vi "niDTS BT INSTR RX Abort.vi"(8 "error in (no error)":errorcluster, 10 "Driver Instance":i32, 11 "niDTS BT INSTR RX in":refnum<class "niDTS BT INSTR RX.lvclass">) -> (0 "error out":errorcluster, 3 "niDTS BT INSTR RX out":refnum<class "niDTS BT INSTR RX.lvclass">)   [LabVIEW 2015, in "niDTS BT.lvlib" / "niDTS BT INSTR RX.lvclass"]
uses:
  niDTS BT INSTR RX.lvclass
  RiviInstDriver/niRfsgBT/Objects/niRfsgBt.lvclass
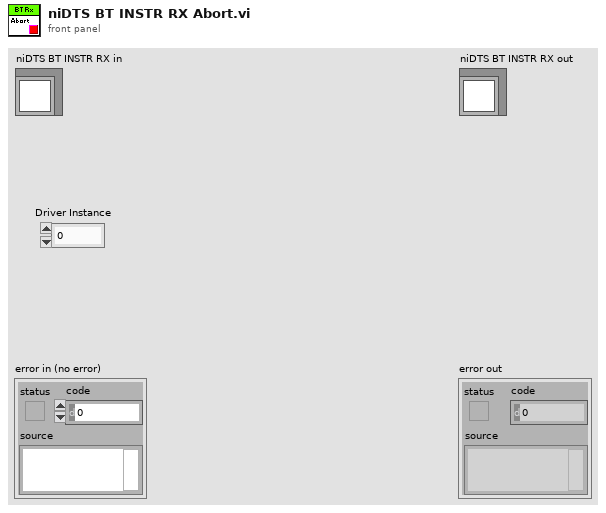
[diagram p1: front panel]
types:
  T1 = typedef "niRfsgBT.lvclass/niRfsgBT INC Handle.ctl" = refnum<data-value>
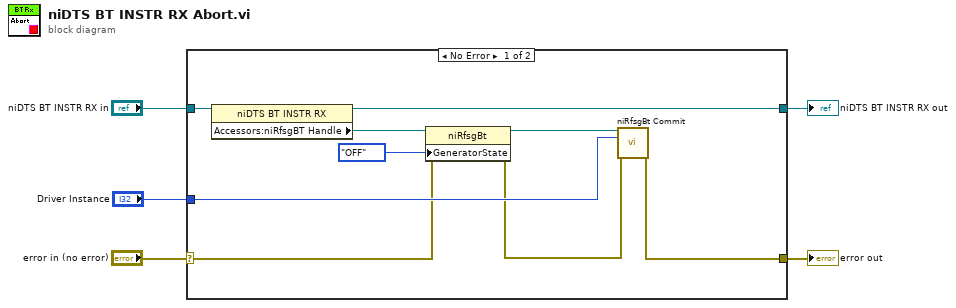
[diagram p0: block diagram]
diagram:
  n1 = case shown="No Error" "error in (no error)" {
    selector: "error in (no error)" -> [w9 w16]
    tunnel: [w7 w16] -> w4
    tunnel: [w12 w15] -> w2
    tunnel: "niDTS BT INSTR RX in" -> [w13 w15]
    tunnel: "Driver Instance" -> [w10 _]
    frame No Error {
      n2 = property class="niDTS BT INSTR RX"(reference=w13) -> (reference out=w12:refnum<class "niDTS BT INSTR RX.lvclass">, "Accessors:niRfsgBT Handle"=w11:T1)  [unwired: 1 in, 1 out]
      n3 = property class="niRfsgBt"(reference=w11, error in=w9, "GeneratorState"=enum16{"OFF", "PENDING", "ON"}."OFF" ("SOURce:RFSG:BLUetooth:GeneratorState")) -> (reference out=w14:T1, error out=w8:errorcluster)
      n4 = call "niRfsgBt Commit.vi"("InstDriver Handle in"=w14, "Instance"=w10, "error in (no error)"=w8) -> ("error out"=w7:errorcluster)  [unwired: 11 in, 1 out]
    }
    frame Error {
    }
  }
  "error out" <- w4
  "niDTS BT INSTR RX out" <- w2
